vi "convert_celsius_fahrenheit.vi"(1 "Celsius":dbl) -> (0 "Fahrenheit":dbl)   [LabVIEW 2013]
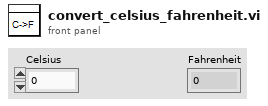
[diagram p1: front panel]
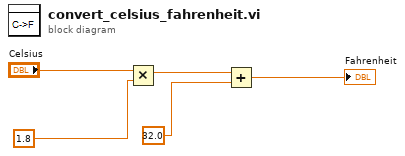
[diagram p0: block diagram]
diagram:
  n1 = Multiply(x="Celsius", y=1.8) -> (x*y=w5:dbl)
  n2 = Add(x=w5, y=32.0) -> (x+y=→"Fahrenheit":dbl)
